vi "Read Access Scope.vi"(8 "error in (no error)":errorcluster, 11 "Attribute.Config in":refnum<class "Attribute.Config.lvclass">) -> (0 "error out":errorcluster, 2 "Access Scope":T1, 3 "Attribute.Config out":refnum<class "Attribute.Config.lvclass">)   [LabVIEW 2019, in "Attribute.Config.lvclass"]
doc: "JKI State Machine Objects (SMO) 1.3.0.56\nJKI - JKI\nCopyright (c) 2017, JKI"
uses:
  Attribute.Config.lvclass
  AccessScope.ctl
  Attribute.Config.lvclass/Attribute.Config.ctl
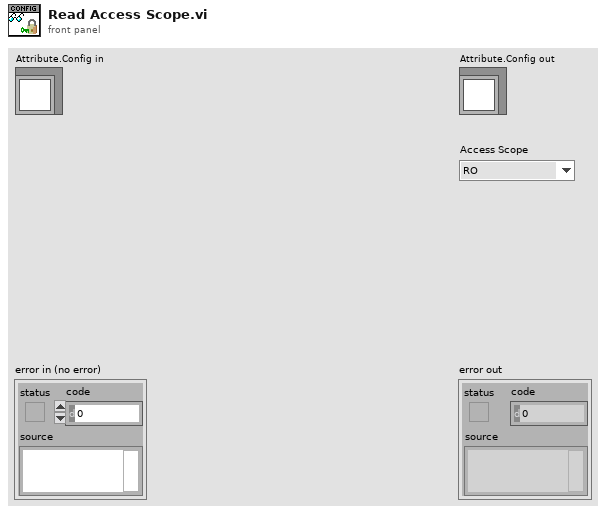
[diagram p1: front panel]
types:
  T1 = typedef "Attribute.Config.lvclass/AccessScope.ctl" = enum16{"RO", "RW"}
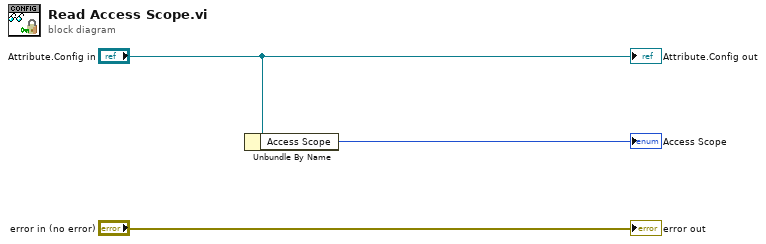
[diagram p0: block diagram]
diagram:
  n1 = Unbundle By Name("Attribute.Config in") -> ("Access Scope"=→"Access Scope":T1)
  "error out" <- "error in (no error)"
  "Attribute.Config out" <- "Attribute.Config in"
